vi "LVFunction_Imop_ModalCoef file_GetInformation.vi"(5 "Coefs file path":path, 11 "error in (no error)":errorcluster) -> (6 "TypePhase":T1, 15 "error out":errorcluster)   [LabVIEW 2018]
uses:
  Controls/WavefrontModalReconstructionType.ctl
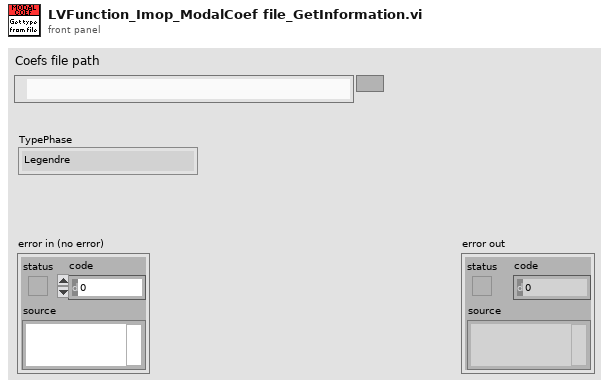
[diagram p1: front panel]
types:
  T1 = typedef "WavefrontModalReconstructionType.ctl" = enum16{"Legendre", "Zernike"}
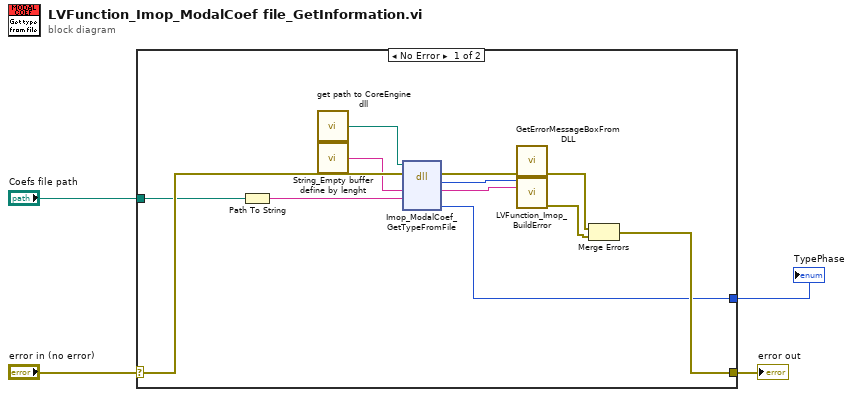
[diagram p0: block diagram]
diagram:
  n1 = case shown="No Error" "error in (no error)" {
    selector: "error in (no error)" -> [w11 w17]
    tunnel: [w10 w17] -> w3
    tunnel: "Coefs file path" -> [w7 _]
    tunnel: [w5 _] -> w1
    frame No Error {
      n2 = Path To String(path=w7) -> (string=w6:string)
      n3 = call "get path to CoreEngine dll.vi"() -> ("path to wavekit library"=w9:path)  [unwired: 14 in, 1 out]
      n4 = call "String_Empty buffer define by lenght.vi"() -> ("Empty buffer"=w8:string)  [unwired: 1 in]
      n5 = dll-call lib="D:/FLE/0.Code/CoreEngine4_Suite/LV2011_interface/DLLs/c_interface_vc100.dll" fn="Imop_ModalCoef_GetTypeFromFile"(path in=w9, error in=w11, "Message"=w8, "Coef file parh"=w6) -> (error out=w16:errorcluster, "return type"=w15:i32, "Message"=w14:string, "type"=w5:u8)  [unwired: 3 in, 1 out]
      n6 = call "GetErrorMessageBoxFromDLL.vi"("error IN"=w16) -> ("error OUT"=w13:errorcluster)  [unwired: 10 in]
      n7 = call "LVFunction_Imop_BuildError.vi"("code"=w15, "String to Prepend to source (\"\")"=w14) -> ("error out"=w12:errorcluster)  [unwired: 13 in]
      n8 = Merge Errors(w13, w12) -> (w10:errorcluster)
    }
    frame Error {
    }
  }
  "error out" <- w3
  "TypePhase" <- w1
